vi "Main.vi"() -> ()   [LabVIEW 2020]
doc: "Run the malleable VI to polymorphic VIs process. The malleable VIs must exist in a single library specified by Source Library Path. When this VI is run, a copy of the library will be placed in Destination Directory, and then each VI in <Source Library Path>\\Polymorphic Templates will be evaluated to determine what polymorphic instance VIs to generate.\n\nAs each polymorphic VI is created, it will be cleaned up (remove the Type Specialization structure and Assert vims), and then the corresponding malleable VI replaced with the new polymorphic VI.\n\nThe resulting library will include a Polymorphic VIs virtual folder containing each polymorphic instance, while the polymorphic VI will be in the same location as the original malleable VI.\n\nThis VI will also update any Call Library Function Node paths that reference a shared library in the lvlib to the shared library in the newly copied lvlib."
panel:
  out "error out":errorcluster
  in  "Destination Directory":path
  in  "Source Library Path (.lvlib)":path
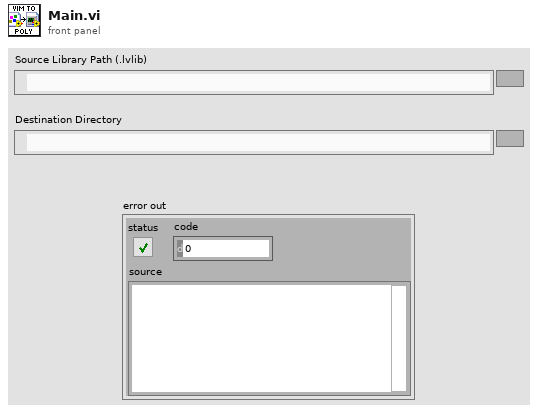
[diagram p1: front panel]
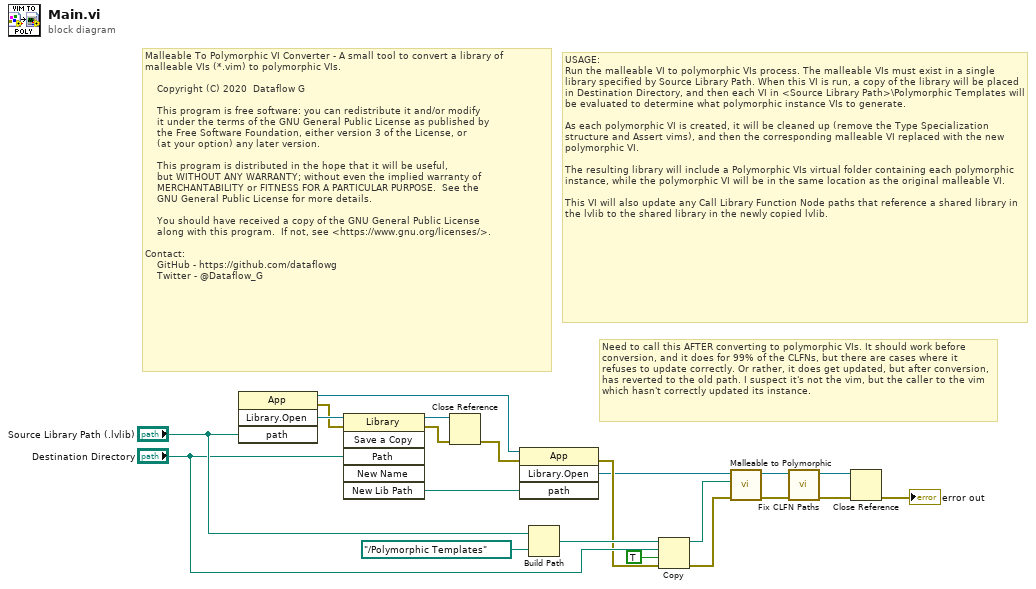
[diagram p0: block diagram]
diagram:
  # "USAGE:\nRun the malleable VI to polymorphic VIs process. The malleable VIs must exist in a single library specified by Source Library Path. When this VI is run, a copy of the library will be placed in Destination Directory, and then each VI in <Source Library Path>\\Polymorphic Templates will be evaluated to determine what polymorphic instance VIs to generate.\n\nAs each polymorphic VI is created, it will be cleaned up (remove the Type Specialization structure and Assert vims), and then the corresponding malleable VI replaced with the new polymorphic VI.\n\nThe resulting library will include a Polymorphic VIs virtual folder containing each polymorphic instance, while the polymorphic VI will be in the same location as the original malleable VI.\n\nThis VI will also update any Call Library Function Node paths that reference a shared library in the lvlib to the shared library in the newly copied lvlib."
  # "Malleable To Polymorphic VI Converter - A small tool to convert a library of malleable VIs (*.vim) to polymorphic VIs.\n\n    Copyright (C) 2020  Dataflow G\n    \n    This program is free software: you can redistribute it and/or modify\n    it under the terms of the GNU General Public License as published by\n    the Free Software Foundation, either version 3 of the License, or\n    (at your option) any later version.\n\n    This program is distributed in the hope that it will be useful,\n    but WITHOUT ANY WARRANTY; without even the implied warranty of\n    MERCHANTABILITY or FITNESS FOR A PARTICULAR PURPOSE.  See the\n    GNU General Public License for more details.\n\n    You should have received a copy of the GNU General Public License\n    along with this program.  If not, see <https://www.gnu.org/licenses/>.\n\nContact:\n    GitHub - https://github.com/dataflowg\n    Twitter - @Dataflow_G"
  # "Need to call this AFTER converting to polymorphic VIs. It should work before conversion, and it does for 99% of the CLFNs, but there are cases where it refuses to update correctly. Or rather, it does get updated, but after conversion, has reverted to the old path. I suspect it's not the vim, but the caller to the vim which hasn't correctly updated its instance."
  n1 = invoke class="App" method="Library.Open"("path"="Source Library Path (.lvlib)") -> (reference out=w9:refnum<vi>, error out=w20:errorcluster, "Open Library"=w21:refnum<vi>)  [unwired: 3 in, 1 out]
  n2 = invoke class="Library" method="Save a Copy"(reference=w21, error in=w20, "Path"="Destination Directory") -> (reference out=w19:refnum<vi>, error out=w18:errorcluster, "New Lib Path"=w17:path)  [unwired: 3 in, 3 out]
  n3 = Close Reference(reference=w19, error in (no error)=w18) -> (error out=w16:errorcluster)
  n4 = invoke class="App" method="Library.Open"(reference=w9, error in=w16, "path"=w17) -> (error out=w7:errorcluster, "Open Library"=w6:refnum<vi>)  [unwired: 1 in, 2 out]
  n5 = Build Path(base path="Source Library Path (.lvlib)", name or relative path=path "../Polymorphic Templates") -> (appended path=w13:path)
  n6 = Copy(8:w7, 9:TRUE ("overwrite (F)"), 10:"Destination Directory", 11:w13) -> (0:w8:errorcluster, 3:w10:path)  [unwired: 2 out]
  n7 = call "Malleable to Polymorphic.vi"("error in (no error)"=w8, "Polymorphic Templates Path"=w10, "Library Ref In"=w6) -> ("error out"=w4:errorcluster, "Library Ref Out"=w5:refnum<vi>)  [unwired: 7 in]
  n8 = call "Fix CLFN Paths.vi"("error in (no error)"=w4, "Library Ref"=w5) -> ("error out"=w3:errorcluster, "Library Ref Out"=w1:refnum<vi>)  [unwired: 8 in]
  n9 = Close Reference(reference=w1, error in (no error)=w3) -> (error out=→"error out":errorcluster)
